vi "set configuration.vi"(8 "error in (no error)":errorcluster, 10 "shm configuration in":refnum<class "Shared Memory configuration.lvclass">, 11 "shared memory editor node in":refnum<class "module editor node.lvclass">) -> (0 "error out":errorcluster, 3 "shared memory editor node out":refnum<class "module editor node.lvclass">)   [LabVIEW 2013, in "Shared Memory editor node.lvclass"]
uses:
  Shared Memory editor node.lvclass
  <vilib>/NI/DCAF/Tag Editor Core/Configuration Editor/Classes/Module editor node/module editor node.lvclass
  module/configuration/Shared Memory configuration.lvclass
  <vilib>/NI/Configuration Framework/serializable configuration/NISE_CEF_serializable configuration.lvclass
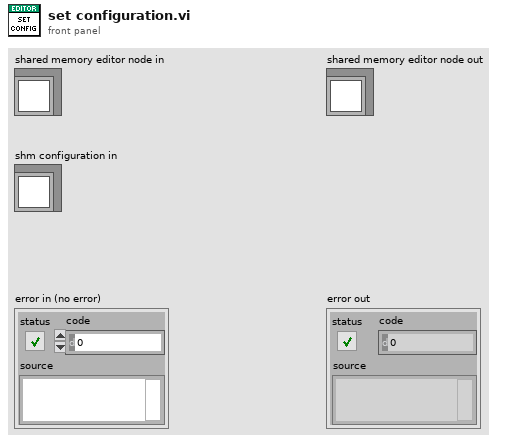
[diagram p1: front panel]
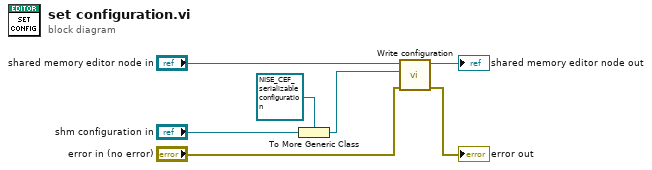
[diagram p0: block diagram]
diagram:
  n1 = To More Generic Class(target class=refnum<class "NISE_CEF_serializable configuration.lvclass"> refnum ("configuration"), reference="shm configuration in") -> (generic class reference=w2:refnum<class "NISE_CEF_serializable configuration.lvclass">)
  n2 = call-dynamic "Write configuration.vi"("error in"="error in (no error)", "configuration"=w2, "NISE_CEF_serializable node in"="shared memory editor node in") -> ("error out"=→"error out":errorcluster, "NISE_CEF_serializable node out"=→"shared memory editor node out":refnum<class "module editor node.lvclass">)  [unwired: 7 in]
